vi "Test Case, MD5 to DBL to MD5.vi"() -> ()   [LabVIEW 2010]
panel:
  out "MD5":string
  in  "error in":errorcluster
  out "error out":errorcluster
  out "all match":bool
  in  "filepath":path=path "C:/5-01-003 Active Electrode Min Max/Waveform 1 -5 mA"
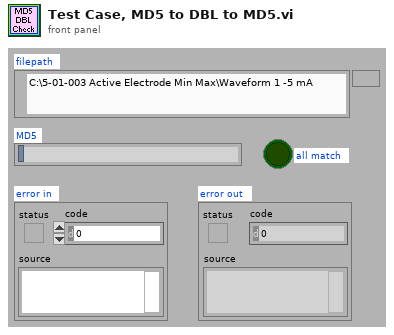
[diagram p1: front panel]
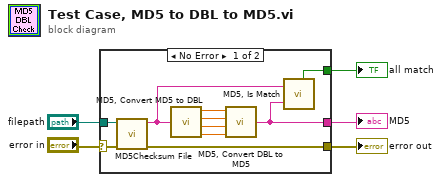
[diagram p0: block diagram]
diagram:
  n1 = case shown="No Error" "error in" {
    selector: "error in" -> [w6 w16]
    tunnel: "filepath" -> [w11 _]
    tunnel: [w9 _] -> w4
    tunnel: [w8 w16] -> w3
    tunnel: [w7 _] -> w1
    frame No Error {
      n2 = call <vilib>:"MD5Checksum File.vi"("error in (no error)"=w6, "Path"=w11) -> ("error out"=w8:errorcluster, "MD5 message-digest"=w10:string)  [unwired: 8 in]
      n3 = call "MD5, Convert MD5 to DBL.vi"("MD5"=w10) -> ("MD5[0]"=w15:dbl, "MD5[1]"=w14:dbl, "MD5[2]"=w13:dbl, "MD5[3]"=w12:dbl)  [unwired: 1 out]
      n4 = call "MD5, Convert DBL to MD5.vi"("MD5[0]"=w15, "MD5[1]"=w14, "MD5[2]"=w13, "MD5[3]"=w12) -> ("MD5"=w7:string)  [unwired: 1 out]
      n5 = call "MD5, Is Match.vi"("MD5(b)"=w7, "MD5(a)"=w10) -> ("MD5 match"=w9:bool)  [unwired: 5 out]
    }
    frame Error {
    }
  }
  "all match" <- w4
  "error out" <- w3
  "MD5" <- w1
